vi "Get Deparment Members.vi"(8 "error in (no error)":errorcluster, 10 "Department(\"\")":string, 11 "CalAttendance in":refnum<class "CalAttendance.lvclass">) -> (0 "error out":errorcluster, 2 "Names(\"\")":string[](array[string]), 3 "CalAttendance out":refnum<class "CalAttendance.lvclass">)   [LabVIEW 2015, in "Admin_Actor.lvlib" / "CalAttendance.lvclass"]
uses:
  CalAttendance.lvclass
  CalAttendance.lvclass/CalAttendance.ctl
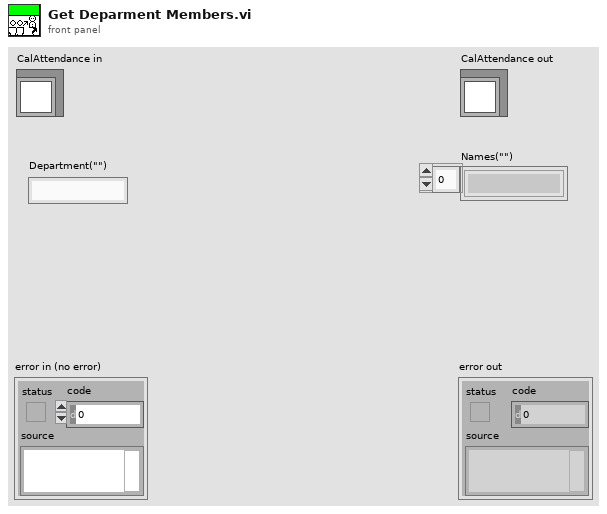
[diagram p1: front panel]
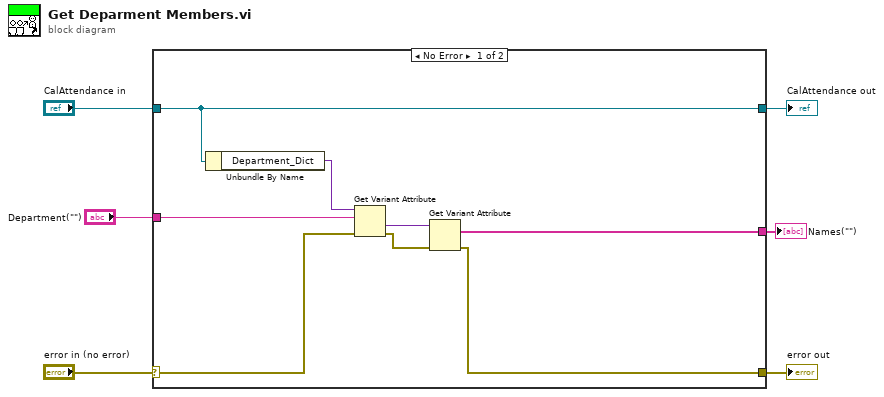
[diagram p0: block diagram]
diagram:
  n1 = case shown="No Error" "error in (no error)" {
    selector: "error in (no error)" -> [w10 w16]
    tunnel: [w7 w16] -> w5
    tunnel: [w14 w15] -> w3
    tunnel: "CalAttendance in" -> [w14 w15]
    tunnel: "Department(\"\")" -> [w12 _]
    tunnel: [w8 _] -> w1
    frame No Error {
      n2 = Unbundle By Name(w14) -> ("Department_Dict"=w13:variant)
      n3 = Get Variant Attribute(Variant=w13, name=w12, error in=w10) -> (value=w11:variant, error out=w9:errorcluster)  [unwired: 1 in, 2 out]
      n4 = Get Variant Attribute(Variant=w11, error in=w9) -> (names=w8:string[], error out=w7:errorcluster)  [unwired: 2 in, 2 out]
    }
    frame Error {
    }
  }
  "error out" <- w5
  "CalAttendance out" <- w3
  "Names(\"\")" <- w1
